vi "Username Input.vi"() -> (3 "Username output":string)   [LabVIEW 2018]
panel:
  in  "More info button":bool
  in  "Cancel button":bool
  in  "Start button":bool
  in  "Username":string
  # "LAG SIM"
  # "Please enter your name for the logbook:"
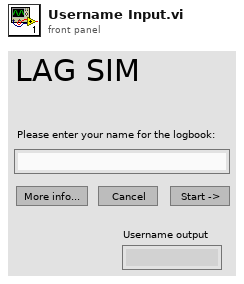
[diagram p1: front panel]
types:
  T1 = enum8{"Enabled", "Disabled", "Disabled and Grayed Out"}
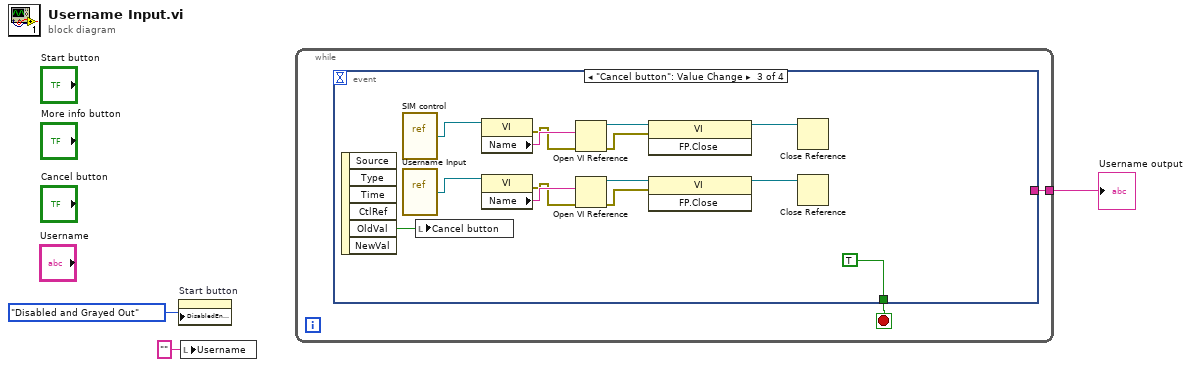
[diagram p0: block diagram]
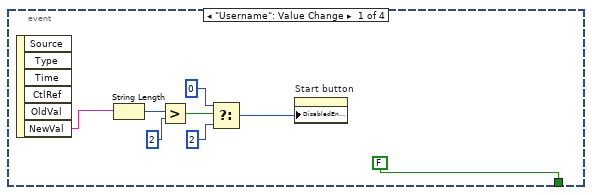
[diagram p2: hidden frame]
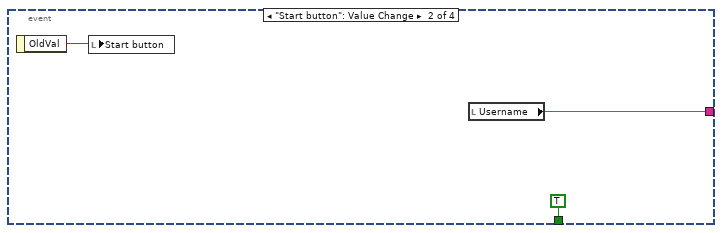
[diagram p3: hidden frame]
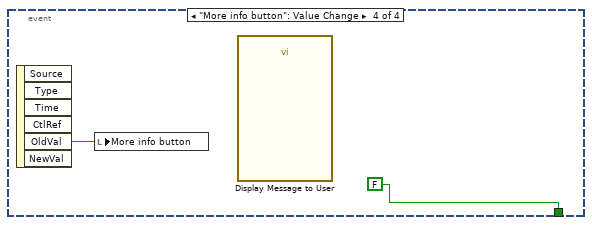
[diagram p4: hidden frame]
diagram:
  n1 = property on="Start button" class="Bool (strict)"("DisabledEnum"=T1."Disabled and Grayed Out" ("Disabled")) -> ()  [unwired: 2 in, 2 out]
  n2 = local write "Username"("" ("Username")) -> ()
  n3 = while {
    tunnel: [w4] -> w1
    stop <- w5 stop-if-true
    n4 = event shown="[2] \"Cancel button\": Value Change" {
      selector: _ -> [_ _ _ _]
      dyn-events: _ -> [_ _ _ _]
      timeout: _ -> [_ _ _ _]
      tunnel: [FALSE TRUE TRUE FALSE] -> w5
      tunnel: [_ w14 _ _] -> w4
      event "Username": Value Change {
        n5 = event-data() -> ("NewVal"=w13:string)  [unwired: 1 in, 5 out]
        n6 = String Length(string=w13) -> (length=w12:i32)
        n7 = Greater?(x=w12, y=2) -> (0:w10:bool)
        n8 = Select(t=0, s=w10, f=2) -> (s? t:f=w6:i32)
        n9 = property on="Start button" class="Bool (strict)"("DisabledEnum"=w6) -> ()  [unwired: 2 in, 2 out]
      }
      event "Start button": Value Change {
        n10 = event-data() -> ("OldVal"=w16:bool)  [unwired: 1 in]
        n11 = local write "Start button"(w16) -> ()
        n12 = local read "Username"() -> (w14:string)
      }
      event "Cancel button": Value Change {
        n13 = event-data() -> ("OldVal"=w30:bool)  [unwired: 1 in, 5 out]
        n14 = vi-ref "SIM control.vi"() -> (w29:refnum<vi>)
        n15 = vi-ref "Username Input.vi"() -> (w22:refnum<vi>)
        n16 = local write "Cancel button"(w30) -> ()
        n17 = property class="VI"(reference=w29) -> (error out=w26:errorcluster, "Name"=w28:string)  [unwired: 1 in, 1 out]
        n18 = property class="VI"(reference=w22) -> (error out=w19:errorcluster, "Name"=w21:string)  [unwired: 1 in, 1 out]
        n19 = Open VI Reference(vi path=w28, error in (no error)=w26) -> (vi reference=w27:refnum<vi>, error out=w25:errorcluster)  [unwired: 4 in]
        n20 = Open VI Reference(vi path=w21, error in (no error)=w19) -> (vi reference=w20:refnum<vi>, error out=w18:errorcluster)  [unwired: 4 in]
        n21 = invoke class="VI" method="FP.Close"(reference=w27, error in=w25) -> (reference out=w24:refnum<vi>)  [unwired: 1 in, 2 out]
        n22 = invoke class="VI" method="FP.Close"(reference=w20, error in=w18) -> (reference out=w17:refnum<vi>)  [unwired: 1 in, 2 out]
        n23 = Close Reference(reference=w24) -> ()  [unwired: 1 in, 1 out]
        n24 = Close Reference(reference=w17) -> ()  [unwired: 1 in, 1 out]
      }
      event "More info button": Value Change {
        n25 = event-data() -> ("OldVal"=w31:bool)  [unwired: 1 in, 5 out]
        n26 = local write "More info button"(w31) -> ()
        n27 = call "Display Message to User"() -> ()  [unwired: 10 in, 2 out]
      }
    }
  }
  "Username output" <- w1
